vi "Scan for Motors.vi"(0 "VISA resource name":refnum<visa-resource-name>, 5 "Starting ID (0)":u8, 7 "Ending ID (253)":u8=253, 9 "Search Timeout (10000 ms)":u32=10000, 11 "error in (no error)":errorcluster) -> (4 "VISA resource name out":refnum<visa-resource-name>, 6 "Motors IDs Found":u8[](array[numeric]), 15 "error out":errorcluster)   [LabVIEW 2016, in "Dynamixel Motor.lvlib"]
doc: "Scans sequentially for motors between <b>Starting ID</b> and <b>Ending ID</b> for no longer than <b>Search Timeout</b>. If all of the motors do not have unique IDs, then motors with duplicate IDs may not be found."
uses:
  Dynamixel Motor.lvlib
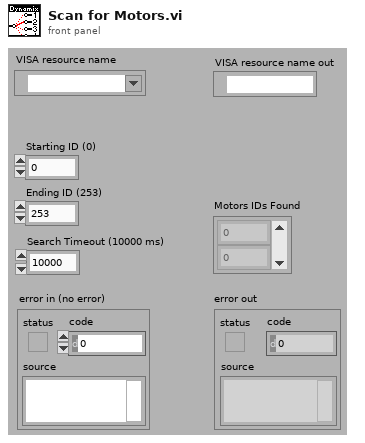
[diagram p1: front panel]
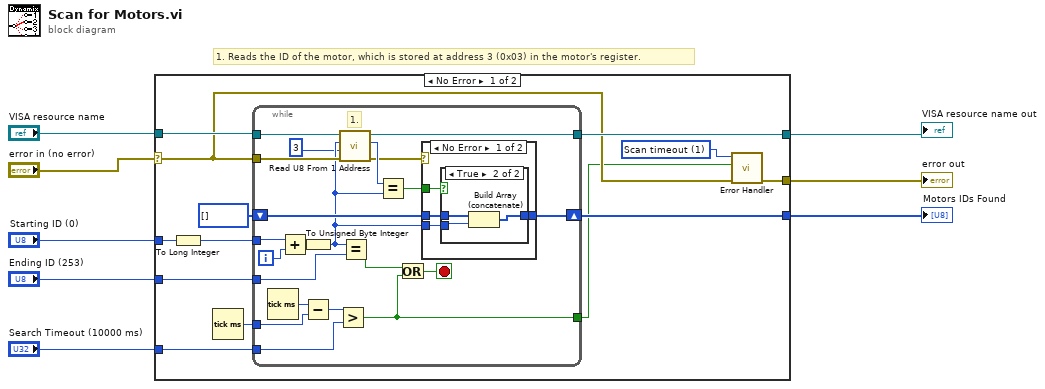
[diagram p0: block diagram]
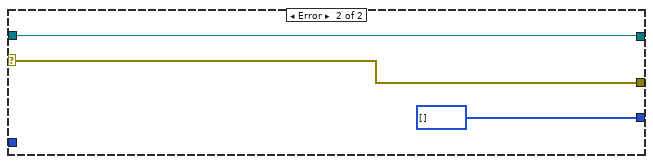
[diagram p4: hidden frame]
diagram:
  # "1. Reads the ID of the motor, which is stored at address 3 (0x03) in the motor's register."
  n1 = case shown="No Error" "error in (no error)" {
    selector: "error in (no error)" -> [w11 w54]
    tunnel: "VISA resource name" -> [w15 w53]
    tunnel: [w21 w53] -> w2
    tunnel: [w12 w54] -> w3
    tunnel: [w17 u8[] []] -> w8
    tunnel: "Starting ID (0)" -> [w20 _]
    tunnel: "Ending ID (253)" -> [w18 _]
    tunnel: "Search Timeout (10000 ms)" -> [w13 _]
    frame No Error {
      w9 = u16 1 items=["Default (no error)", "Scan timeout", "Invalid motor checksum", "Unexpected return string", "Invalid address range"] ("Error type")
      n2 = To Long Integer(number=w20) -> (32bit integer=w16:i32)
      n3 = Tick Count (ms)() -> (millisecond timer value=w14:u32)
      n4 = while {
        tunnel: w15 -> [w41]
        shift-right: [w37] -> w17
        shift-left: u8[] [] -> [w39]
        tunnel: [w35] -> w21
        tunnel: w11 -> [w34]
        tunnel: w16 -> [w33]
        tunnel: w18 -> [w32]
        tunnel: w14 -> [w25]
        tunnel: w13 -> [w23]
        tunnel: [w22] -> w10
        i -> [w42]
        stop <- w36 stop-if-true
        # "1."
        n5 = Tick Count (ms)() -> (millisecond timer value=w26:u32)
        n6 = Add(x=w33, y=w42) -> (x+y=w38:i32)
        n7 = To Unsigned Byte Integer(number=w38) -> (unsigned 8bit integer=w29:u8)
        n8 = Subtract(x=w26, y=w25) -> (x-y=w24:u32)
        n9 = Greater?(x=w24, y=w23) -> (0:w22:bool)
        n10 = call "Read U8 From 1 Address.vi"("Error in (no error)"=w34, "Address number (0)"=u8 3, "Motor ID (0)"=w29, "VISA resource name"=w41) -> ("error out"=w27:errorcluster, "Data"=w31:u8, "VISA resource name out"=w35:refnum<visa-resource-name>)  [unwired: 5 in]
        n11 = Equal?(x=w29, y=w32) -> (x = y?=w30:bool)
        n12 = Equal?(x=w31, y=w29) -> (x = y?=w40:bool)
        n13 = Or(x=w30, y=w22) -> (x .or. y?=w36:bool)
        n14 = case shown="No Error" w27 {
          tunnel: w40 -> [w46 _]
          tunnel: w39 -> [w45 w51]
          tunnel: [w44 w51] -> w37
          tunnel: w29 -> [w43 _]
          frame No Error {
            n15 = case shown="True" w46 {
              tunnel: w45 -> [w47 w50]
              tunnel: w43 -> [_ w49]
              tunnel: [w47 w48] -> w44
              frame False {
              }
              frame True {
                n16 = Build Array (concatenate)(w50, w49) -> (w48:u8[])
              }
            }
          }
          frame Error {
          }
        }
      }
      n17 = call "Error Handler.vi"("error in (no error)"=w11, "Error? (no error)"=w10, "Error type"=w9) -> ("error out"=w12:errorcluster)  [unwired: 8 in]
    }
    frame Error {
    }
  }
  "Motors IDs Found" <- w8
  "error out" <- w3
  "VISA resource name out" <- w2
